vi "Instrument Name Create.vi"(1 "Instrument Type":string, 2 "Model":string, 3 "Manufacturer":string) -> (0 "Name":string)   [LabVIEW 2021]
uses:
  NML Data Acq Globals.vi
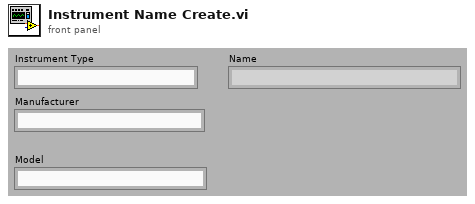
[diagram p1: front panel]
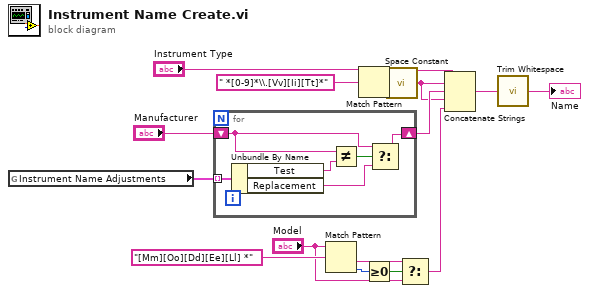
[diagram p0: block diagram]
diagram:
  n1 = global read "NML Data Acq Globals.vi" "Instrument Name Adjustments"() -> (w2:cluster{"Test":string, "Replacement":string}[])
  n2 = for {
    shift-right: [w17] -> w11
    shift-left: "Manufacturer" -> [w16]
    tunnel: w2 -> [w21] mode=indexing
    n3 = Unbundle By Name(w21) -> ("Test"=w20:string, "Replacement"=w18:string)
    n4 = Not Equal?(x=w16, y=w20) -> (x != y?=w19:bool)
    n5 = Select(t=w16, s=w19, f=w18) -> (s? t:f=w17:string)
  }
  n6 = Match Pattern(string="Model", regular expression="[Mm][Oo][Dd][Ee][Ll] *" ("search string/char (-)")) -> (after substring=w3:string, offset past match=w7:i32)  [unwired: 1 in, 2 out]
  n7 = Match Pattern(string="Instrument Type", regular expression=" *[0-9]*\\.[Vv][Ii][Tt]*" ("search string/char (-)")) -> (before substring=w13:string)  [unwired: 1 in, 3 out]
  n8 = Greater Or Equal To 0?(x=w7) -> (x >= 0?=w6:bool)
  n9 = call <vilib>:"Space Constant.vi"() -> ("String"=w10:string)
  n10 = Select(t=w3, s=w6, f="Model") -> (s? t:f=w5:string)
  n11 = Concatenate Strings(w13, w10, w11, w10, w5) -> (w12:string)
  n12 = call <vilib>:"Trim Whitespace.vi"("string"=w12) -> ("trimmed string"=→"Name":string)  [unwired: 1 in]
